vi "Set initial.vi"(8 "error in (no error)":errorcluster, 10 "Circuit cluster":T1, 11 "G-UE in":refnum<class "G-UE.lvclass">) -> (0 "error out":errorcluster, 3 "G-UE out":refnum<class "G-UE.lvclass">)   [LabVIEW 2016, in "G-UE.lvclass"]
uses:
  G-UE.lvclass
  TypeDefs/Circuit Cluster.ctl
  GateAbst/GateAbst.lvclass
  G-UE.lvclass/G-UE.ctl
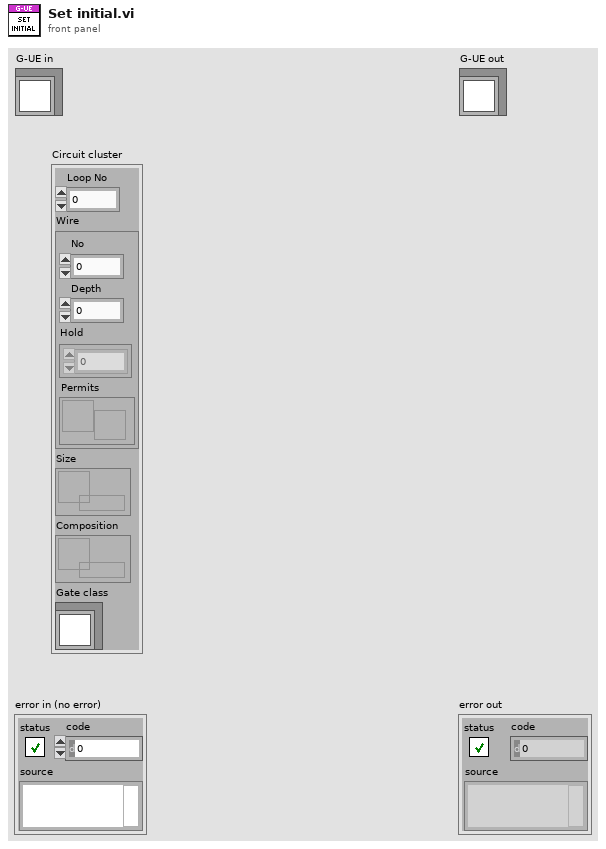
[diagram p1: front panel]
types:
  T1 = typedef "Circuit Cluster.ctl" = cluster{"Loop No":i32, "Wire":cluster{"No":i32, "Depth":i32, "Hold":i32[][], "Permits":refnum<notifier>}, "Size":refnum<queue>, "Composition":refnum<queue>, "Gate class":refnum<class "GateAbst.lvclass">}
  T2 = typedef "NI_Matrix.lvlib/ComplexMatrix.ctl" = cdb[][]
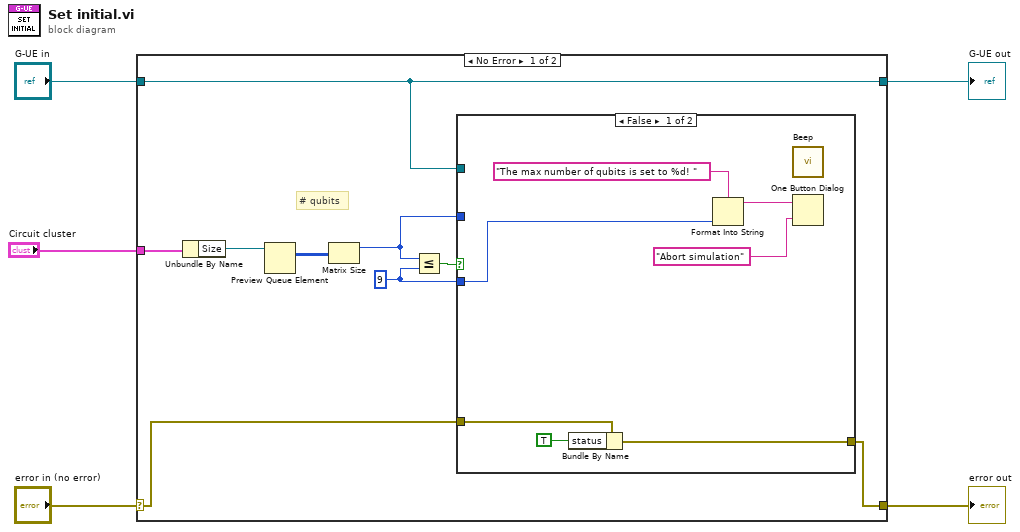
[diagram p0: block diagram]
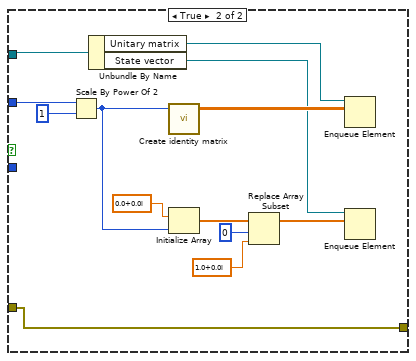
[diagram p2: hidden frame]
diagram:
  n1 = case shown="No Error" "error in (no error)" {
    selector: "error in (no error)" -> [w7 w36]
    tunnel: [w6 w36] -> w4
    tunnel: [w14 w35] -> w2
    tunnel: "G-UE in" -> [w14 w35]
    tunnel: "Circuit cluster" -> [w12 _]
    frame No Error {
      w10 = 9 ("y")
      # "# qubits"
      n2 = Unbundle By Name(w12) -> ("Size"=w13:refnum<queue>)
      n3 = Preview Queue Element(queue=w13) -> (element=w9:i32[][])  [unwired: 2 in, 3 out]
      n4 = Matrix Size(0:w9) -> (1:w8:i32)  [unwired: 1 out]
      n5 = Less Or Equal?(x=w8, y=w10) -> (x <= y?=w11:bool)
      n6 = case shown="False" w11 {
        tunnel: w14 -> [_ w33]
        tunnel: w8 -> [_ w23]
        tunnel: w10 -> [w19 _]
        tunnel: w7 -> [w16 w22]
        tunnel: [w15 w22] -> w6
        frame False {
          n7 = Bundle By Name(cluster=w16, "status"=TRUE) -> (w15:errorcluster)
          n8 = Format Into String(format string="The max number of qubits is set to %d! " ("message"), w19) -> (resulting string=w18:string)  [unwired: 2 in, 1 out]
          n9 = call <vilib>:"Beep.vi"() -> ()  [unwired: 12 in]
          n10 = One Button Dialog(message=w18, button name ("OK")="Abort simulation") -> ()  [unwired: 1 out]
        }
        frame True {
          n11 = Scale By Power Of 2(n=w23, x=1) -> (x*2^n=w26:i32)
          n12 = Unbundle By Name(w33) -> ("Unitary matrix"=w32:refnum<queue>, "State vector"=w25:refnum<queue>)
          n13 = call "Create identity matrix.vi"("Matrix size"=w26) -> ("Identity Matrix"=w31:T2)  [unwired: 4 in]
          n14 = Initialize Array(cdb 0.0+0.0i ("element"), w26) -> (w28:cdb[])
          n15 = Replace Array Subset(array=w28, new element=cdb 1.0+0.0i ("element"), index=0) -> (w24:cdb[])
          n16 = Enqueue Element(queue=w32, element=w31) -> ()  [unwired: 2 in, 3 out]
          n17 = Enqueue Element(queue=w25, element=w24) -> ()  [unwired: 2 in, 3 out]
        }
      }
    }
    frame Error {
    }
  }
  "error out" <- w4
  "G-UE out" <- w2
